vi "hw3.5.vi"() -> ()   [LabVIEW 2014]
panel:
  out "reaction time":u32
  in  "Stop Timer":bool
  out "state":string
  in  "stop program":bool
  out "LED":bool
  in  "Start Button":bool
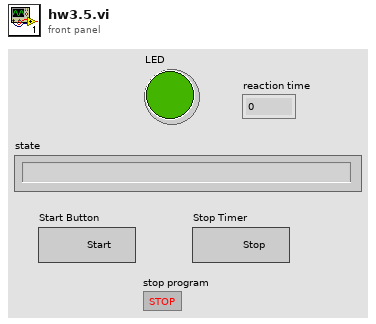
[diagram p1: front panel]
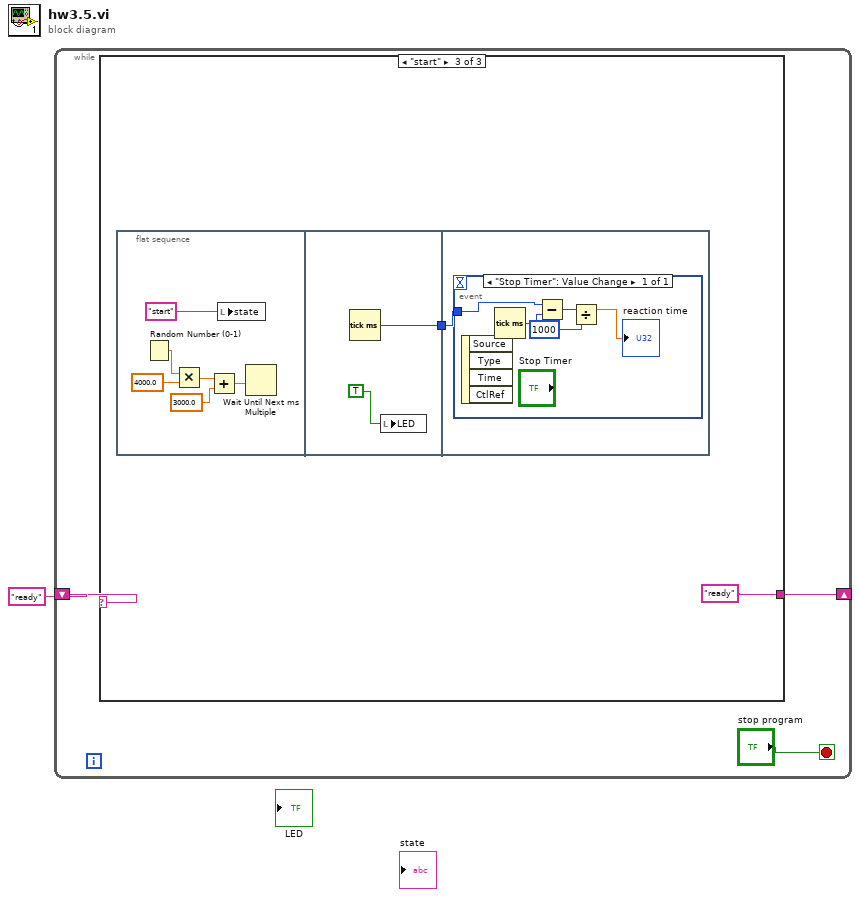
[diagram p0: block diagram]
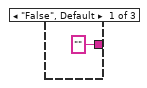
[diagram p2: hidden frame]
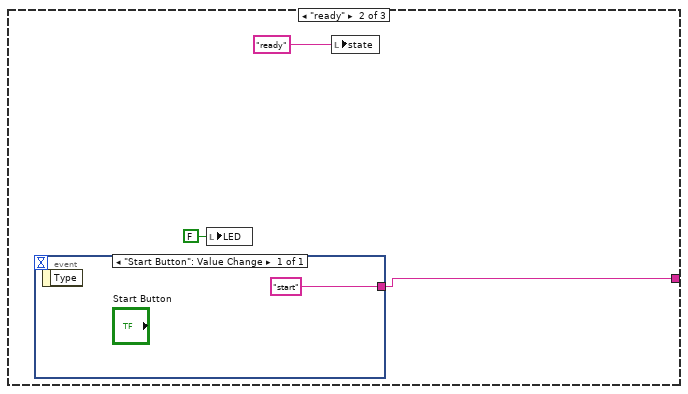
[diagram p3: hidden frame]
diagram:
  n1 = while {
    shift-right: [w3] -> _
    shift-left: "ready" -> [w4]
    stop <- "stop program" stop-if-true
    n2 = case shown="\"start\"" w4 {
      tunnel: ["" w8 "ready"] -> w3
      frame "False", Default {
      }
      frame "ready" {
        n3 = event shown="[0] \"Start Button\": Value Change" {
          selector: _ -> [_]
          dyn-events: _ -> [_]
          timeout: _ -> [_]
          tunnel: ["start"] -> w8
          event "Start Button": Value Change {
            n4 = event-data() -> ()  [unwired: 1 in, 1 out]
          }
        }
        n5 = local write "LED"(FALSE ("LED")) -> ()
        n6 = local write "state"("ready" ("User Instructions")) -> ()
      }
      frame "start" {
        n7 = flat-sequence {
          tunnel: [w18] -> w10
          tunnel: w10 -> [w20]
          frame #0 {
            n8 = Random Number (0-1)() -> (number: 0 to 1=w17:dbl)
            n9 = Multiply(x=w17, y=4000.0) -> (x*y=w15:dbl)
            n10 = Add(x=w15, y=3000.0) -> (x+y=w13:dbl)
            n11 = local write "state"("start" ("User Instructions")) -> ()
            n12 = Wait Until Next ms Multiple(millisecond multiple=w13) -> ()  [unwired: 1 out]
          }
          frame #1 {
            n13 = Tick Count (ms)() -> (millisecond timer value=w18:u32)
            n14 = local write "LED"(TRUE ("LED")) -> ()
          }
          frame #2 {
            n15 = event shown="[0] \"Stop Timer\": Value Change" {
              selector: _ -> [_]
              dyn-events: _ -> [_]
              timeout: _ -> [_]
              tunnel: w20 -> [w24]
              event "Stop Timer": Value Change {
                n16 = event-data() -> ()  [unwired: 1 in, 4 out]
                n17 = Tick Count (ms)() -> (millisecond timer value=w25:u32)
                n18 = Subtract(x=w24, y=w25) -> (x-y=w23:u32)
                n19 = Divide(x=w23, y=u32 1000) -> (x/y=→"reaction time":dbl)
              }
            }
          }
        }
      }
    }
  }
